vi "Configure Job.vi"(8 "error in (no error)":errorcluster, 10 "JSON String":string) -> (0 "error out":errorcluster, 3 "Job out":refnum<class "Job.lvclass">)   [LabVIEW 2014, in "Job.lvclass"]
uses:
  Job.lvclass
  Controls/Job Parameters - STYP.ctl
  Job.lvclass/Job.ctl
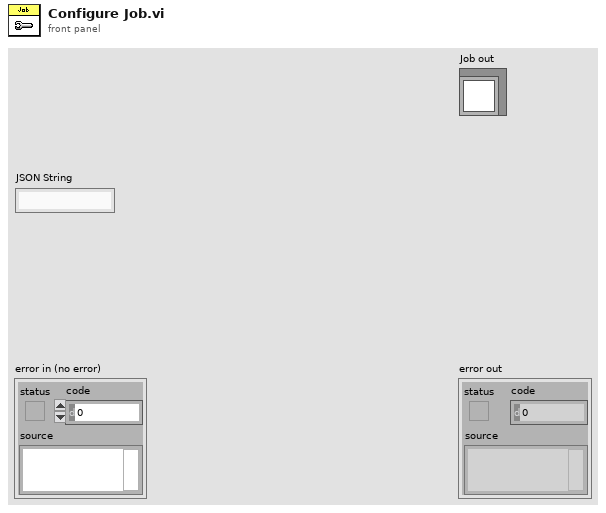
[diagram p1: front panel]
types:
  T1 = typedef "Job Parameters - STYP.ctl" = cluster{"Executor_Number":string, "Workspace_Path":string}
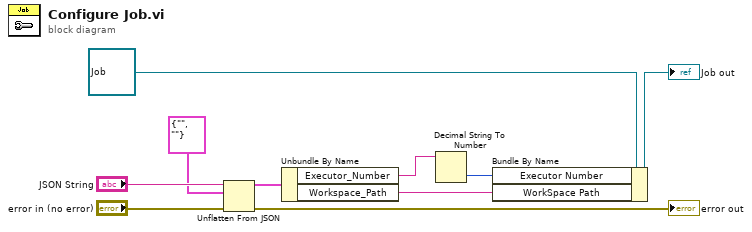
[diagram p0: block diagram]
diagram:
  n1 = Unflatten From JSON(JSON string="JSON String", type and defaults=T1 {"Executor_Number"="", "Workspace_Path"=""} ("Job_Param"), error in (no error)="error in (no error)") -> (value=w3:T1, error out=→"error out":errorcluster)  [unwired: 4 in]
  n2 = Unbundle By Name(w3) -> ("Executor_Number"=w4:string, "Workspace_Path"=w2:string)
  n3 = Decimal String To Number(string=w4) -> (number=w1:i32)  [unwired: 2 in, 1 out]
  n4 = Bundle By Name(cluster=refnum<class "Job.lvclass"> refnum ("Job in"), "Executor Number"=w1, "WorkSpace Path"=w2) -> (→"Job out":refnum<class "Job.lvclass">)
